vi "GA Set Trap Prm Single.vi"(6 "dSmoothTime":i16, 7 "dVelStart":dbl, 8 "error in (no error)":errorcluster caption="错误输入（无错误）", 9 "dDec":dbl, 10 "dAcc":dbl, 11 "nAxisNum":i16) -> (0 "error out":errorcluster caption="错误输出", 3 "function return":i32)   [LabVIEW 2024, in "GAS.lvlib"]
doc: "extern \"C\" __declspec(dllimport) int GA_SetTrapPrmSingle(short nAxisNum,double dAcc,double dDec,double dVelStart,short dSmoothTime);"
uses:
  GAS.lvlib
  GAS.dll
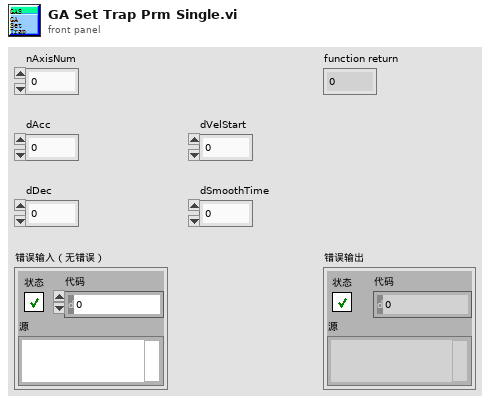
[diagram p1: front panel]
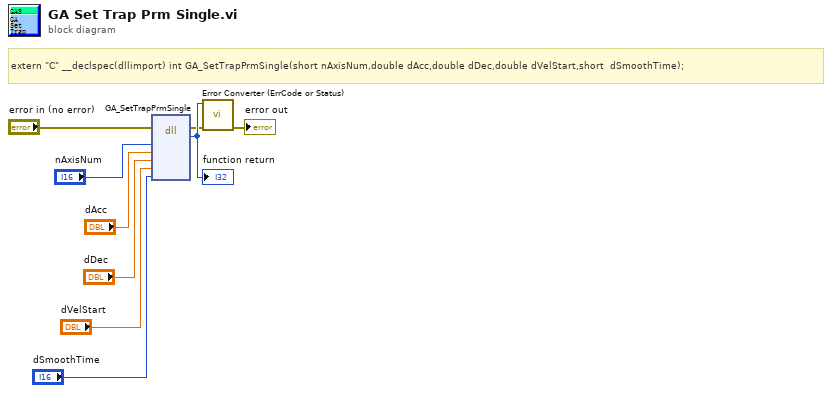
[diagram p0: block diagram]
diagram:
  # "extern \"C\" __declspec(dllimport) int GA_SetTrapPrmSingle(short nAxisNum,double dAcc,double dDec,double dVelStart,short  dSmoothTime);"
  n1 = dll-call lib="PTH2?abs D实验室软件（勿删）集成测试系统GAS.*" fn="GA_SetTrapPrmSingle"(error in="error in (no error)", "nAxisNum"="nAxisNum", "dAcc"="dAcc", "dDec"="dDec", "dVelStart"="dVelStart", "dSmoothTime"="dSmoothTime") -> (error out=w2:errorcluster, w9:i32)  [unwired: 7 in, 1 out]
  "function return" <- w9
  n2 = call "Error Converter (ErrCode or Status).vi"("error in (no error)"=w2, "error code"=w9) -> ("error out"=→"error out":errorcluster)  [unwired: 9 in]
